vi "WriteData (DDT).vi"(6 "value index (0)":u64, 7 "DDT":dynamicdata(waveform), 8 "error in (no error)":errorcluster, 9 "channel index (0)":u32, 10 "operation (0: create)":T2(ring)=enum."Create", 11 "Excel refnum":T1) -> (0 "error out":errorcluster, 3 "Excel refnum out":T1)   [LabVIEW 2017, in "NI_ExcelFile.lvlib"]
uses:
  <vilib>/express/express shared/NI_ExcelFile/NI_ExcelFile.lvlib
  <vilib>/express/express shared/NI_ExcelFile/Ctrls/ExcelRefnum.ctl
  <vilib>/express/express shared/NI_ExcelFile/Ctrls/MainData.ctl
  <vilib>/express/express shared/NI_ExcelFile/Ctrls/StreamMode.ctl
  <vilib>/express/express shared/NI_ExcelFile/Ctrls/TimeColumnMode.ctl
  <vilib>/express/express shared/NI_ExcelFile/Ctrls/FileAttribute.ctl
  <vilib>/express/express shared/NI_ExcelFile/Ctrls/Columns.ctl
  <vilib>/express/express shared/NI_ExcelFile/Ctrls/ColumnInfo.ctl
  <vilib>/express/express shared/NI_ExcelFile/Ctrls/DataType.ctl
  <vilib>/express/express shared/NI_ExcelFile/Ctrls/wd_recordInfo.ctl
  <vilib>/express/express shared/NI_ExcelFile/Ctrls/disk_TemplateFile.ctl
  <vilib>/express/express shared/NI_ExcelFile/Ctrls/meta_file.ctl
  <vilib>/express/express shared/NI_ExcelFile/Ctrls/meta_Block.ctl
  <vilib>/express/express shared/NI_ExcelFile/Ctrls/meta_BlockType.ctl
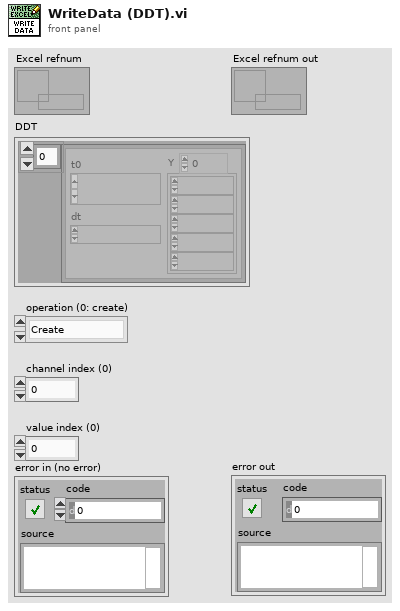
[diagram p1: front panel]
types:
  T1 = typedef "NI_ExcelFile.lvlib/ExcelRefnum.ctl" = refnum<data-value>
  T2 = enum16{"Append values", "Create", "Replace values at index", "Replace all values"}
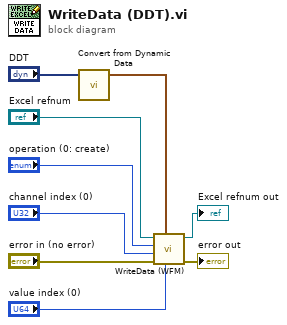
[diagram p0: block diagram]
diagram:
  n1 = call "Convert from Dynamic Data"("Dynamic Data Type"="DDT") -> ("Waveform"=w6:waveform(dbl))  [unwired: 3 in]
  n2 = call <vilib>:"WriteData (WFM).vi"("value index (0)"="value index (0)", "WFM"=w6, "error in (no error)"="error in (no error)", "channel index (0)"="channel index (0)", "operation (0: create)"="operation (0: create)", "Excel refnum"="Excel refnum") -> ("error out"=→"error out":errorcluster, "Excel refnum out"=→"Excel refnum out":T1)  [unwired: 4 in]
